vi "Set UUT Info.vi"(0 "reference in":refnum<class "UUT.lvclass">, 1 "Part Number":string, 2 "Upper Push Limit (lb)":dbl, 3 "Lower Pull Limit (lb)":dbl, 4 "Lower Push Limit (lb)":dbl, 5 "Upper Pull Limit (lb)":dbl, 7 "error in (no error)":errorcluster, 9 "Push Position (mm)":dbl, 11 "Pull Position (mm)":dbl) -> (20 "reference out":refnum<class "UUT.lvclass">, 27 "error out":errorcluster)   [LabVIEW 2017, in "UUT.lvclass"]
uses:
  UUT.lvclass
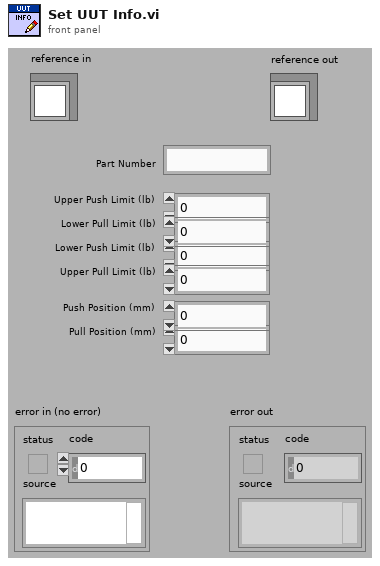
[diagram p1: front panel]
types:
  T1 = typedef "UUT.lvclass/ObjectAttributes.ctl" = cluster{"UUT Info":cluster{"Part Number":string, "Lower Push Limit (lb)":dbl, "Upper Push Limit (lb)":dbl, "Lower Pull Limit (lb)":dbl, "Upper Pull Limit (lb)":dbl, "Push Position (mm)":dbl, "Pull Position (mm)":dbl}, "Test Results":cluster{"Test Time":timestamp, "Number of Trials":u32, "Push Values (lb)":dbl[], "Push Average (lb)":dbl, "Push Std Dev (lb)":dbl, "Push Passed":bool, "Pull Values (lb)":dbl[], "Pull Average (lb)":dbl, "Pull Std Dev (lb)":dbl, "Pull Passed":bool}}
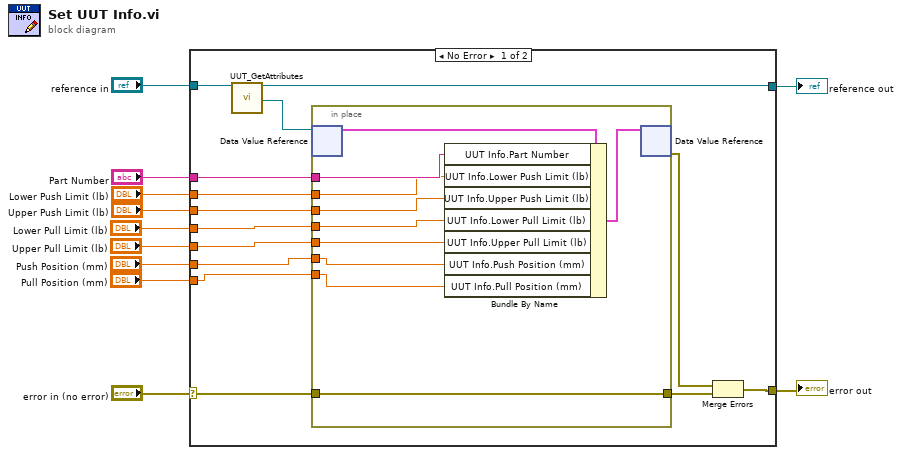
[diagram p0: block diagram]
diagram:
  n1 = case shown="No Error" "error in (no error)" {
    selector: "error in (no error)" -> [w15 w37]
    tunnel: [w22 w37] -> w10
    tunnel: [w23 w36] -> w8
    tunnel: "reference in" -> [w25 w36]
    tunnel: "Part Number" -> [w20 _]
    tunnel: "Lower Push Limit (lb)" -> [w19 _]
    tunnel: "Upper Push Limit (lb)" -> [w18 _]
    tunnel: "Lower Pull Limit (lb)" -> [w17 _]
    tunnel: "Upper Pull Limit (lb)" -> [w16 _]
    tunnel: "Push Position (mm)" -> [w13 _]
    tunnel: "Pull Position (mm)" -> [w12 _]
    frame No Error {
      n2 = call "UUT_GetAttributes.vi"("reference in"=w25) -> ("reference out"=w23:refnum<class "UUT.lvclass">, "DataRef"=w21:refnum<data-value>)  [unwired: 15 in, 2 out]
      n3 = in-place {
        in-place-border: w20 -> [w33]
        in-place-border: w19 -> [w32]
        in-place-border: w18 -> [w31]
        in-place-border: w17 -> [w30]
        in-place-border: w16 -> [w29]
        in-place-border: [w28] -> w14
        in-place-border: w15 -> [w28]
        in-place-border: w13 -> [w27]
        in-place-border: w12 -> [w26]
        n4 = in-place-dvr #1(w21) -> (w34:T1)  [unwired: 1 out]
        n5 = Bundle By Name(cluster=w34, "UUT Info.Part Number"=w33, "UUT Info.Lower Push Limit (lb)"=w32, "UUT Info.Upper Push Limit (lb)"=w31, "UUT Info.Lower Pull Limit (lb)"=w30, "UUT Info.Upper Pull Limit (lb)"=w29, "UUT Info.Push Position (mm)"=w27, "UUT Info.Pull Position (mm)"=w26) -> (w35:T1)
        n6 = in-place-dvr #1(w35) -> (w24:errorcluster)  [unwired: 1 out]
      }
      n7 = Merge Errors(w24, w14) -> (w22:errorcluster)
    }
    frame Error {
    }
  }
  "error out" <- w10
  "reference out" <- w8
